vi "global_stop_calibration.vi"() -> ()   [LabVIEW 2015]
panel:
  in  "stop":bool
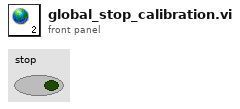
[diagram p1: front panel]
diagram:
